vi "Load Custom Waveform.vi"() -> (2 "Waveform Created?":bool, 3 "Output Waveform":waveform(dbl))   [LabVIEW 2021]
uses:
  <vilib>/Utility/file.llb/Read Delimited Spreadsheet (string).vi
panel:
  in  "File Type":enum32{"CSV", "TDMS", "TDM"}(radio)
  in  "Read From":i32 caption="Read From Row/Wfm Index" min=0
  in  "Load File":bool
  in  "Suggest Naming?":bool=TRUE
  in  "Waveform Name":string
  in  "Cancel":bool
  in  "OK":bool
  out "Actual Sample Size":i32
  out "Actual Duration (s)":dbl format="%#_6p"
  out "Waveform Preview":waveform(dbl)(graph)
  in  "Sample Rate (Hz)":dbl=10000000.0 min=0.0 format="%#_6p"
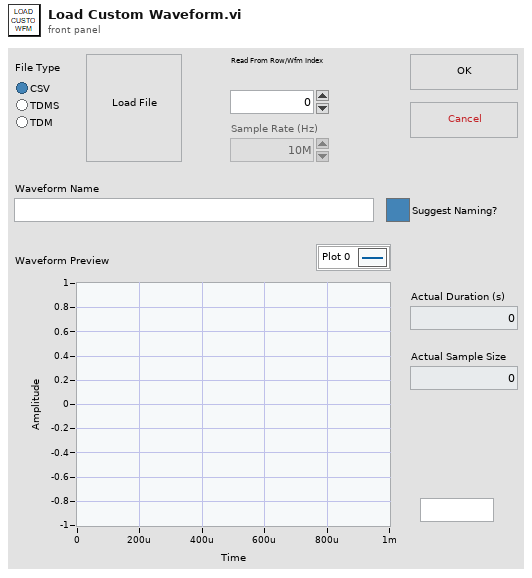
[diagram p1: front panel]
types:
  T1 = cluster{"pattern (all files)":string, "pattern label":string, "prompt":string}
  T2 = enum16{"Ready", "Update Wfm", "Suggest Name Update"}
  T3 = cluster{"pattern (all files)":string, "pattern label":string, "prompt":string}[]
  T4 = enum8{"Enabled", "Disabled", "Disabled and Grayed Out"}
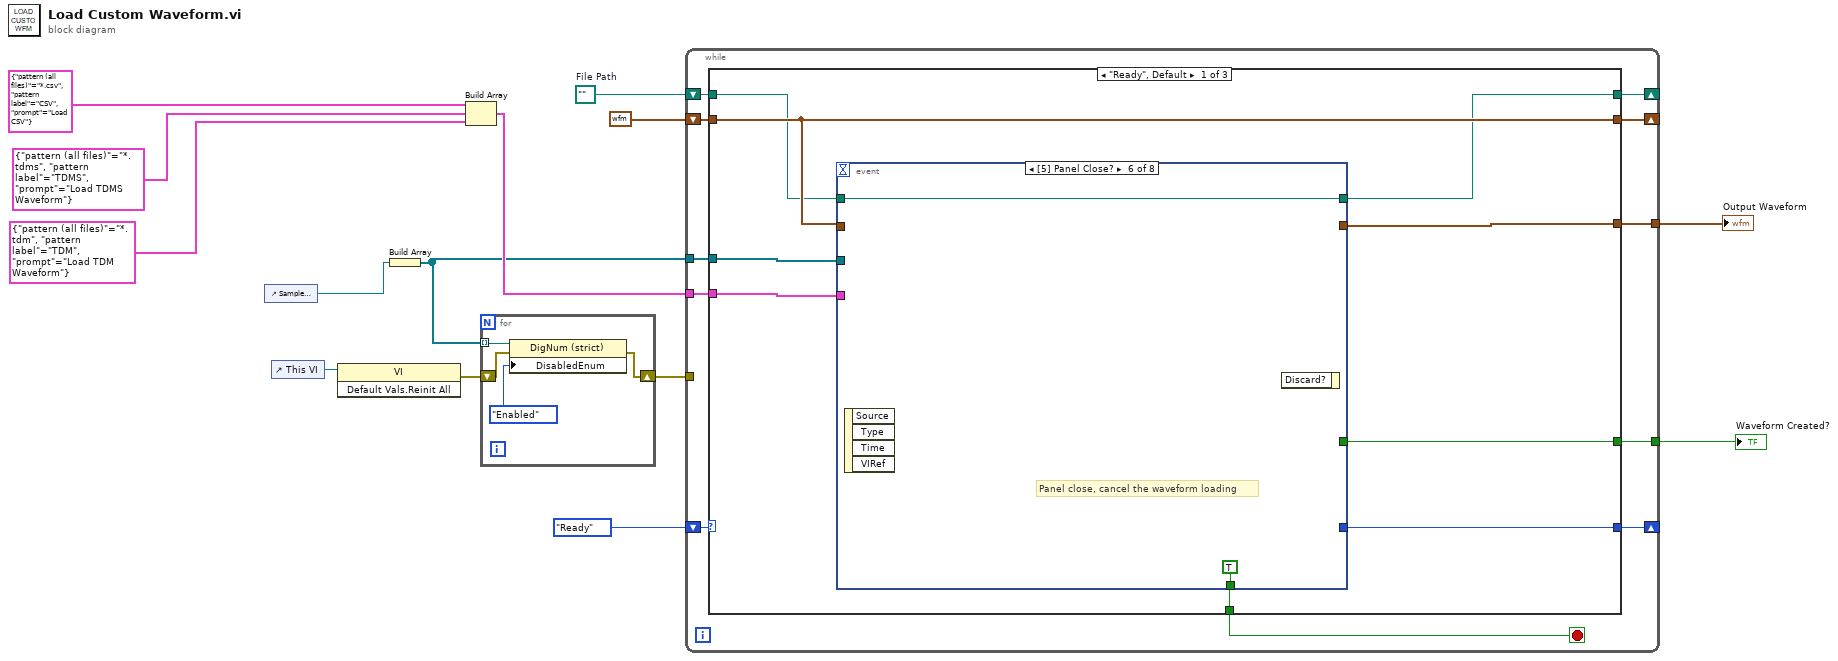
[diagram p0: block diagram]
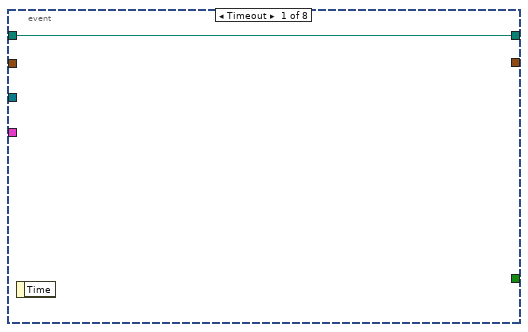
[diagram p2: hidden frame]
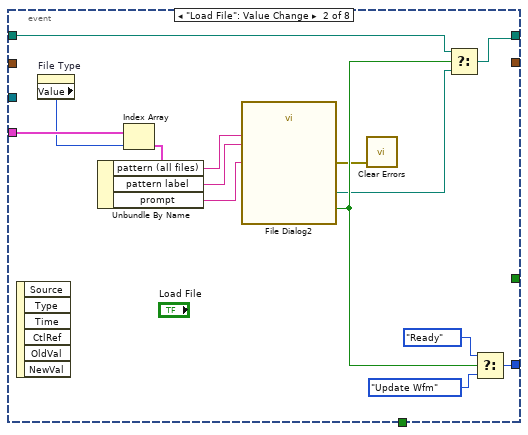
[diagram p3: hidden frame]
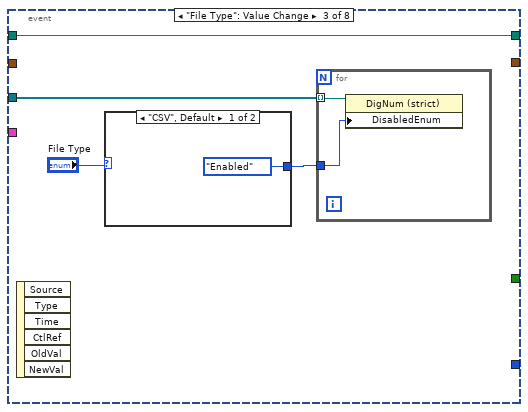
[diagram p4: hidden frame]
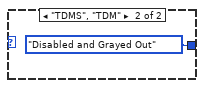
[diagram p5: hidden frame]
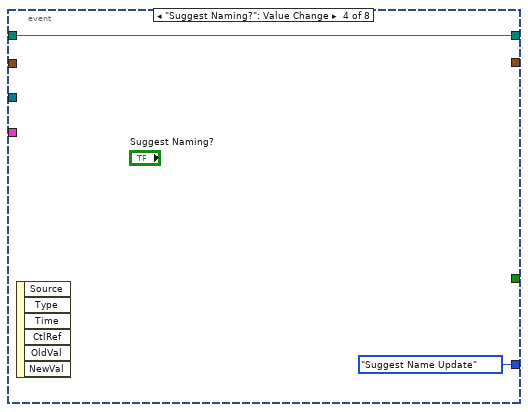
[diagram p6: hidden frame]
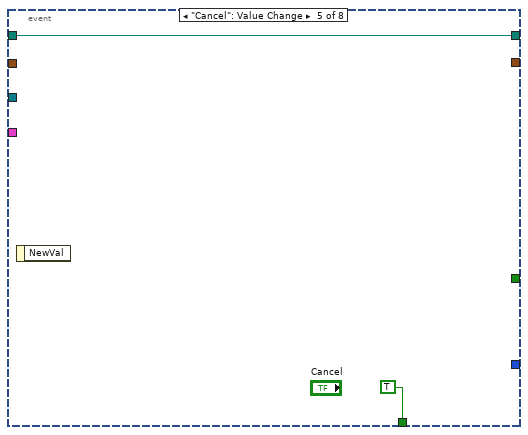
[diagram p7: hidden frame]
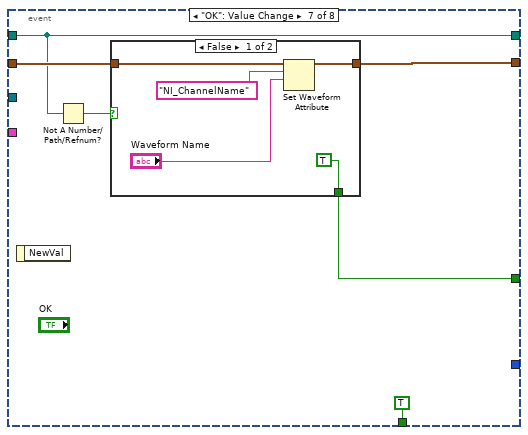
[diagram p8: hidden frame]
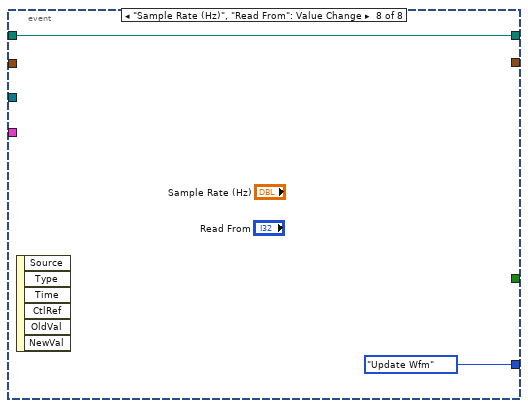
[diagram p10: hidden frame]
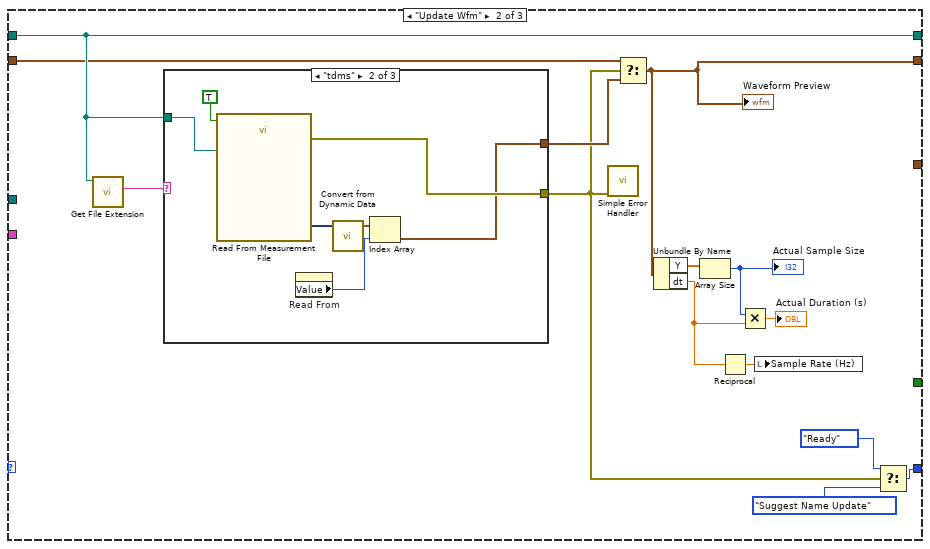
[diagram p11: hidden frame]
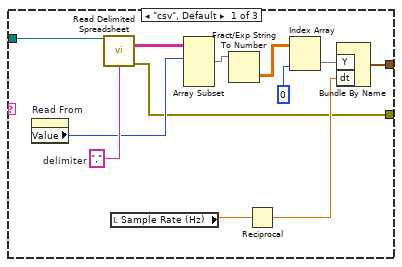
[diagram p12: hidden frame]
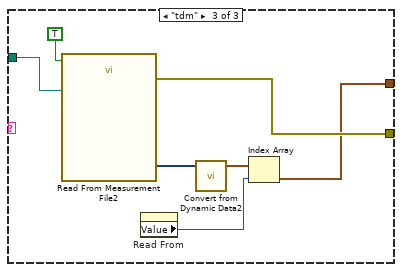
[diagram p13: hidden frame]
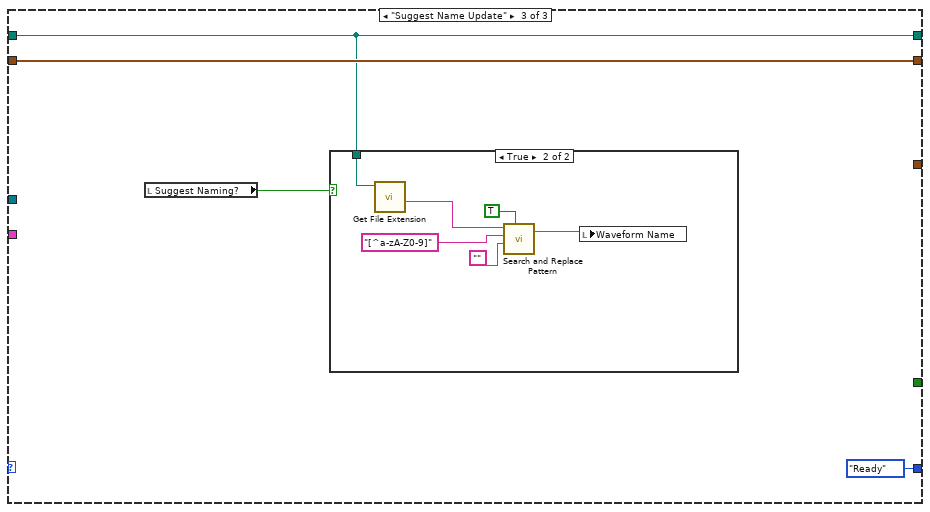
[diagram p14: hidden frame]
diagram:
  w12 = path ""  # File Path
  n1 = control-ref of="Sample Rate (Hz)"() -> (w8:refnum<vi>)
  n2 = control-ref of="This VI"() -> (w9:refnum<vi>)
  n3 = invoke class="VI" method="Default Vals.Reinit All"(reference=w9) -> (error out=w7:errorcluster)  [unwired: 2 in, 2 out]
  n4 = Build Array(w8) -> (w2:refnum<vi>[])
  n5 = Build Array(T1 {"pattern (all files)"="*.csv", "pattern label"="CSV", "prompt"="Load CSV"}, T1 {"pattern (all files)"="*.tdms", "pattern label"="TDMS", "prompt"="Load TDMS Waveform"}, T1 {"pattern (all files)"="*.tdm", "pattern label"="TDM", "prompt"="Load TDM Waveform"}) -> (w3:T3)
  n6 = for {
    tunnel: w2 -> [w18] mode=indexing
    shift-right: [w15] -> w6
    shift-left: w7 -> [w16]
    n7 = property class="DigNum (strict)"(reference=w18, error in=w16, "DisabledEnum"=T4."Enabled" ("Disabled")) -> (error out=w15:errorcluster)  [unwired: 1 out]
  }
  n8 = while {
    tunnel: [w28] -> w14
    shift-right: [w26] -> _
    shift-left: T2."Ready" -> [w27]
    shift-right: [w24] -> _
    shift-left: w12 -> [w25]
    shift-right: [w22] -> _
    shift-left: waveform(dbl) {"t0"=timestamp(0 s since 1904-01-01), "dt"=1.0, "Y"=[]} ("Output Waveform") -> [w23]
    tunnel: [w21] -> w10
    tunnel: w6 -> [_]
    tunnel: w3 -> [w20]
    tunnel: w2 -> [w19]
    stop <- w29 stop-if-true
    n9 = case shown="\"Ready\", Default" w27 {
      tunnel: [w38 _ _] -> w29
      tunnel: [w37 _ _] -> w28
      tunnel: [w36 w90 T2."Ready"] -> w26
      tunnel: w25 -> [w33 w93 w122]
      tunnel: [w32 w93 w122] -> w24
      tunnel: w23 -> [w35 w92 w124]
      tunnel: [w35 w86 w124] -> w22
      tunnel: [w34 _ _] -> w21
      tunnel: w20 -> [w31 _ _]
      tunnel: w19 -> [w30 _ _]
      frame "Ready", Default {
        n10 = event shown="[5] Panel Close?" {
          selector: _ -> [_ _ _ _ _ _ _ _]
          dyn-events: _ -> [_ _ _ _ _ _ _ _]
          timeout: _ -> [_ _ _ _ _ _ _ _]
          tunnel: [_ _ _ _ TRUE TRUE TRUE _] -> w38
          tunnel: [_ _ _ _ _ _ w68 _] -> w37
          tunnel: [_ w52 _ T2."Suggest Name Update" _ _ _ T2."Update Wfm"] -> w36
          tunnel: w35 -> [_ _ _ _ _ _ w72 _]
          tunnel: [_ _ _ _ _ _ w71 _] -> w34
          tunnel: w33 -> [w39 w49 w57 w62 w64 w67 w69 w79]
          tunnel: [w39 w47 w57 w62 w64 w67 w69 w79] -> w32
          tunnel: w31 -> [_ w46 _ _ _ _ _ _]
          tunnel: w30 -> [_ _ w56 _ _ _ _ _]
          event Timeout {
            n11 = event-data() -> ()  [unwired: 1 in, 1 out]
          }
          event "Load File": Value Change {
            n12 = event-data() -> ()  [unwired: 1 in, 6 out]
            n13 = property on="File Type" class="RadioBtnsControl (strict)"() -> ("Value"=w41:enum32{"CSV", "TDMS", "TDM"})  [unwired: 2 in, 2 out]
            n14 = Index Array(array=w46, index=w41) -> (element=w45:T1)
            n15 = Unbundle By Name(w45) -> ("pattern (all files)"=w44:string, "pattern label"=w43:string, "prompt"=w42:string)
            n16 = call "File Dialog2"("prompt"=w42, "pattern (all files)"=w44, "pattern label"=w43) -> ("selected path"=w48:path, "cancelled"=w50:bool, "error out"=w40:errorcluster)  [unwired: 9 in, 1 out]
            n17 = call <vilib>:"Clear Errors.vi"("error in (no error)"=w40) -> ()  [unwired: 5 in, 2 out]
            n18 = Select(t=w49, s=w50, f=w48) -> (s? t:f=w47:path)
            n19 = Select(t=T2."Ready", s=w50, f=T2."Update Wfm") -> (s? t:f=w52:T2)
          }
          event "File Type": Value Change {
            n20 = event-data() -> ()  [unwired: 1 in, 6 out]
            n21 = case shown="\"CSV\", Default" "File Type" {
              tunnel: [T4."Enabled" ("Disabled") T4."Disabled and Grayed Out" ("Disabled")] -> w55
              frame "CSV", Default {
              }
              frame "TDMS", "TDM" {
              }
            }
            n22 = for {
              tunnel: w56 -> [w61] mode=indexing
              tunnel: w55 -> [w60]
              n23 = property class="DigNum (strict)"(reference=w61, "DisabledEnum"=w60) -> ()  [unwired: 1 in, 2 out]
            }
          }
          event "Suggest Naming?": Value Change {
            n24 = event-data() -> ()  [unwired: 1 in, 6 out]
          }
          event "Cancel": Value Change {
            n25 = event-data() -> ()  [unwired: 1 in, 1 out]
          }
          event Panel Close? {
            # "Panel close, cancel the waveform loading"
            n26 = event-data() -> ()  [unwired: 1 in, 4 out]
            n27 = event-data() -> ()  [unwired: 2 in, 1 out]
          }
          event "OK": Value Change {
            n28 = event-data() -> ()  [unwired: 1 in, 1 out]
            n29 = Not A Number/Path/Refnum?(number/path/refnum=w69) -> (NaN/Path/Refnum?=w70:bool)
            n30 = case shown="False" w70 {
              tunnel: w72 -> [w78 _]
              tunnel: [w75 _] -> w71
              tunnel: [TRUE _] -> w68
              frame False {
                n31 = Set Waveform Attribute(5:"Waveform Name", 6:"NI_ChannelName" ("name"), 7:w78) -> (3:w75:waveform(dbl))  [unwired: 1 in, 2 out]
              }
              frame True {
              }
            }
          }
          event "Sample Rate (Hz)", "Read From": Value Change {
            n32 = event-data() -> ()  [unwired: 1 in, 6 out]
          }
        }
      }
      frame "Update Wfm" {
        n33 = call <vilib>:"Get File Extension.vi"("file"=w93) -> ("lowercase file extension"=w94:string)  [unwired: 6 in, 4 out]
        n34 = case shown="\"tdms\"" w94 {
          tunnel: w93 -> [w105 w113 w120]
          tunnel: [w96 w109 w116] -> w91
          tunnel: [w95 w112 w119] -> w89
          frame "csv", Default {
            w106 = ","  # delimiter
            n35 = property on="Read From" class="DigNum (strict)"() -> ("Value"=w100:i32)  [unwired: 2 in, 2 out]
            n36 = call-poly <vilib>:"Read Delimited Spreadsheet.vi"("file path (dialog if empty)"=w105, "delimiter (\\t)"=w106) -> ("all rows"=w101:string[][], "error out"=w95:errorcluster)  [unwired: 8 in, 4 out]
            n37 = local read "Sample Rate (Hz)"() -> (w103:dbl)
            n38 = Array Subset(array=w101, index (row)=w100) -> (w99:string[][])  [unwired: 3 in]
            n39 = Fract/Exp String To Number(string=w99) -> (number=w98:dbl[][])  [unwired: 3 in, 1 out]
            n40 = Reciprocal(x=w103) -> (1/x=w102:dbl)
            n41 = Index Array(array=w98, index (col)=0) -> (element=w97:dbl[])  [unwired: 1 in]
            n42 = Bundle By Name("Y"=w97, "dt"=w102) -> (w96:waveform(dbl))  [unwired: 1 in]
          }
          frame "tdms" {
            n43 = call "Read From Measurement File"("Filename"=w113, "Reset"=TRUE) -> ("error out"=w112:errorcluster, "Signals"=w111:dynamicdata)  [unwired: 4 in, 4 out]
            n44 = property on="Read From" class="DigNum (strict)"() -> ("Value"=w108:i32)  [unwired: 2 in, 2 out]
            n45 = call "Convert from Dynamic Data"("Dynamic Data Type"=w111) -> ("Array of Waveform"=w110:waveform(dbl)[])  [unwired: 3 in]
            n46 = Index Array(array=w110, index=w108) -> (element=w109:waveform(dbl))
          }
          frame "tdm" {
            n47 = call "Read From Measurement File2"("Filename"=w120, "Reset"=TRUE) -> ("error out"=w119:errorcluster, "Signals"=w118:dynamicdata)  [unwired: 4 in, 4 out]
            n48 = property on="Read From" class="DigNum (strict)"() -> ("Value"=w115:i32)  [unwired: 2 in, 2 out]
            n49 = call "Convert from Dynamic Data2"("Dynamic Data Type"=w118) -> ("Array of Waveform"=w117:waveform(dbl)[])  [unwired: 3 in]
            n50 = Index Array(array=w117, index=w115) -> (element=w116:waveform(dbl))
          }
        }
        n51 = call <vilib>:"Simple Error Handler.vi"("error in (no error)"=w89) -> ()  [unwired: 4 in, 5 out]
        n52 = Select(t=w92, s=w89, f=w91) -> (s? t:f=w86:waveform(dbl))
        "Waveform Preview" <- w86
        n53 = Unbundle By Name(w86) -> ("Y"=w85:dbl[], "dt"=w82:dbl)
        n54 = Array Size(array=w85) -> (size(s)=w83:i32)
        "Actual Sample Size" <- w83
        n55 = Reciprocal(x=w82) -> (1/x=w81:dbl)
        n56 = Multiply(x=w83, y=w82) -> (x*y=→"Actual Duration (s)":dbl)
        n57 = local write "Sample Rate (Hz)"(w81) -> ()
        n58 = Select(t=T2."Ready", s=w89, f=T2."Suggest Name Update") -> (s? t:f=w90:T2)
      }
      frame "Suggest Name Update" {
        n59 = local read "Suggest Naming?"() -> (w123:bool)
        n60 = case shown="True" w123 {
          tunnel: w122 -> [_ w130]
          frame False {
          }
          frame True {
            n61 = call <vilib>:"Get File Extension.vi"("file"=w130) -> ("filename without extension"=w128:string)  [unwired: 6 in, 4 out]
            n62 = call <vilib>:"Search and Replace Pattern.vi"("string"=w128, "regular expression (\"\")"="[^a-zA-Z0-9]" ("regular expression"), "replace string (\"\")"="" ("replace string (\"\")"), "replace all? (F)"=TRUE) -> ("result string"=w125:string)  [unwired: 1 in, 1 out]
            n63 = local write "Waveform Name"(w125) -> ()
          }
        }
      }
    }
  }
  "Waveform Created?" <- w14
  "Output Waveform" <- w10
